vi "2_3.vi"() -> ()   [LabVIEW 2010]
panel:
  out "Таблиця 2 - Результат":string[][](table)
  in  "Сортувати стовпчик":dbl
  in  "Таблиця 1 - Вхідні дані":string[][](table)
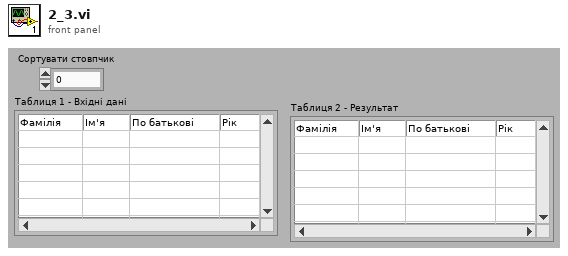
[diagram p1: front panel]
types:
  T1 = cluster{"[0]":string, "[1]":string, "[2]":string, "[3]":string, "[4]":string, "[5]":string, "[6]":string, "[7]":string, "[8]":string}
  T2 = cluster{"[0]":string, "[1]":string, "[2]":string, "[3]":string, "[4]":string, "[5]":string, "[6]":string, "[7]":string, "[8]":string}[]
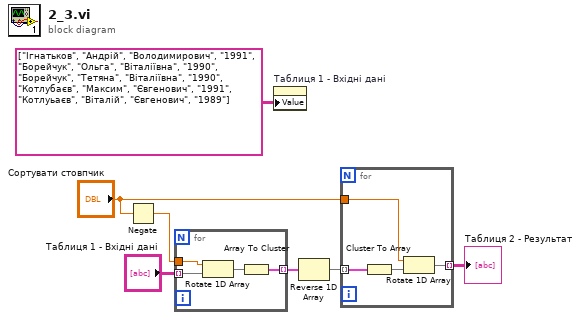
[diagram p0: block diagram]
diagram:
  n1 = Negate(x="Сортувати стовпчик") -> (-x=w3:dbl)
  n2 = for {
    tunnel: [w11] -> w5 mode=indexing
    tunnel: "Таблиця 1 - Вхідні дані" -> [w9] mode=indexing
    tunnel: w3 -> [w8]
    n3 = Rotate 1D Array(1:w9, 2:w8) -> (0:w10:string[])
    n4 = Array To Cluster(array=w10) -> (cluster=w11:T1)
  }
  n5 = property on="Таблиця 1 - Вхідні дані" class="Tbl (strict)"("Value"=string[][] [["Ігнатьков", "Андрій", "Володимирович", "1991"], ["Борейчук", "Ольга", "Віталіївна", "1990"], ["Борейчук", "Тетяна", "Віталіївна", "1990"], ["Котлубаєв", "Максим", "Євгенович", "1991"], ["Котлуьаєв", "Віталій", "Євгенович", "1989"]] ("Таблиця 1")) -> ()  [unwired: 2 in, 2 out]
  n6 = Reverse 1D Array(array=w5) -> (reversed array=w6:T2)
  n7 = for {
    tunnel: w6 -> [w14] mode=indexing
    tunnel: "Сортувати стовпчик" -> [w13]
    tunnel: [w12] -> w1 mode=indexing
    n8 = Cluster To Array(cluster=w14) -> (array=w15:string[])
    n9 = Rotate 1D Array(1:w15, 2:w13) -> (0:w12:string[])
  }
  "Таблиця 2 - Результат" <- w1
